vi "List All Elements.vi"(8 "error in (no error)":errorcluster, 10 "Filter App Credentials (F)":bool, 11 "OAuthAccessToken in":refnum<class "OAuthAccessToken.lvclass">) -> (0 "error out":errorcluster, 1 "Values":string[](array[string]), 2 "Keys":string[](array[string]), 3 "OAuthAccessToken out":refnum<class "OAuthAccessToken.lvclass">)   [LabVIEW 2013, in "OAuthAccessToken.lvclass"]
uses:
  OAuthAccessToken.lvclass
  OAuthAccessToken.lvclass/OAuthAccessToken.ctl
  OAuth2 Token Element -- enum.ctl
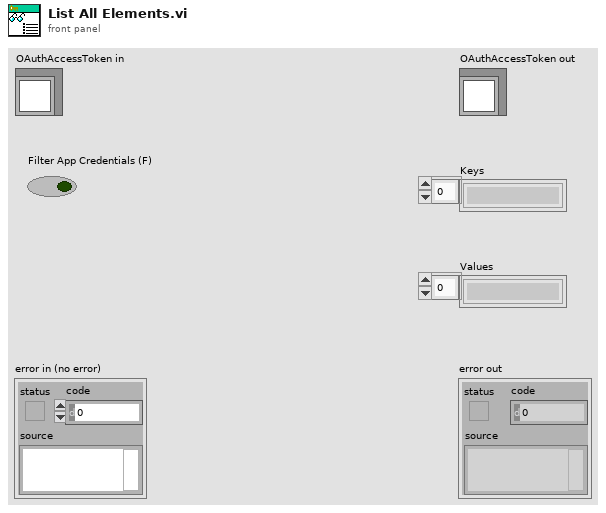
[diagram p1: front panel]
types:
  T1 = typedef "OAuthAccessToken.lvclass/OAuth2 Token Element -- enum.ctl" = enum16{"client_id", "client_secret", "response_type", "scope", "redirect_uri", "error", "error_description", "error_uri", "grant_type", "code", "access_token", "token_type", "expires_in", "username", "password", "refresh_token", "endpoint element"}
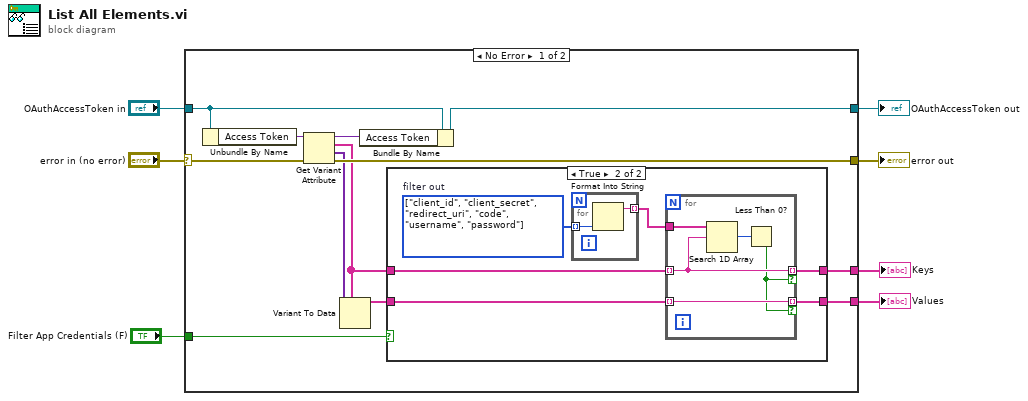
[diagram p0: block diagram]
diagram:
  n1 = case shown="No Error" "error in (no error)" {
    selector: "error in (no error)" -> [w17 w36]
    tunnel: [w16 w36] -> w6
    tunnel: [w18 w35] -> w4
    tunnel: "OAuthAccessToken in" -> [w19 w35]
    tunnel: [w11 _] -> w3
    tunnel: [w10 _] -> w2
    tunnel: "Filter App Credentials (F)" -> [w12 _]
    frame No Error {
      n2 = Unbundle By Name(w19) -> ("Access Token"=w15:variant)
      n3 = Get Variant Attribute(Variant=w15, error in=w17) -> (duplicate Variant=w14:variant, names=w8:string[], values=w13:variant[], error out=w16:errorcluster)  [unwired: 2 in]
      n4 = Variant To Data(type=w8, Variant=w13) -> (data=w9:string[])  [unwired: 1 in, 1 out]
      n5 = Bundle By Name(cluster=w19, "Access Token"=w14) -> (w18:refnum<class "OAuthAccessToken.lvclass">)
      n6 = case shown="True" w12 {
        tunnel: [w20 w24] -> w11
        tunnel: [w21 w23] -> w10
        tunnel: w9 -> [w21 w22]
        tunnel: w8 -> [w20 w26]
        frame False {
        }
        frame True {
          w27 = T1[] [enum."client_id", enum."client_secret", enum."redirect_uri", enum."code", enum."username", enum."password"] items=["client_id", "client_secret", "response_type", "scope", "redirect_uri", "error", "error_description", "error_uri", "grant_type", "code", "access_token", "token_type", "expires_in", "username", "password", "refresh_token", "endpoint element"]  # filter out
          n7 = for {
            tunnel: w27 -> [w34] mode=indexing
            tunnel: [w33] -> w25 mode=indexing
            n8 = Format Into String(w34) -> (resulting string=w33:string)  [unwired: 3 in, 1 out]
          }
          n9 = for {
            tunnel: w26 -> [w30] mode=indexing
            tunnel: w25 -> [w32]
            tunnel: [w30] -> w24 mode=indexing if=w28
            tunnel: [w29] -> w23 mode=indexing if=w28
            tunnel: w22 -> [w29] mode=indexing
            n10 = Search 1D Array(1D array=w32, element=w30) -> (index of element=w31:i32)  [unwired: 1 in]
            n11 = Less Than 0?(x=w31) -> (x < 0?=w28:bool)
          }
        }
      }
    }
    frame Error {
    }
  }
  "error out" <- w6
  "OAuthAccessToken out" <- w4
  "Keys" <- w3
  "Values" <- w2
